vi "Check Posttrigger Countdown.vi"(8 "error in (no error)":errorcluster, 11 "Triggered Log in":refnum<class "Triggered Log.lvclass">) -> (0 "error out":errorcluster, 3 "Triggered Log out":refnum<class "Triggered Log.lvclass">)   [LabVIEW 2012, in "Triggered Log.lvclass"]
doc: "If the log is currently in the Posttrigger state, this VI checks the posttrigger countdown to see if it has reached zero. If so, this VI sets the triggered state of the log to either Waiting on Trigger or Complete based on whether the start trigger is retriggerable. It also notifies any listeners of the changed trigger state. Finally, if the posttrigger countdown is complete, this VI flushes any remaining data in the log buffer and closes the current file instance if specified."
uses:
  Triggered Log.lvclass
  Triggered Log.lvclass/Triggered Log.ctl
  Triggered Log State.ctl
  Engine/Classes/Logs/Segmented Logs/Segmented Log/Segmented Log.lvclass/Segmented Log.ctl
  Shared/Classes/Log File Specifications/Log File Specification/Log File Specification.lvclass/Log File Specification.ctl
  Flush Buffer Data to File.vi
  On Triggered Log State Change.vi
  Flush Buffer Data.vi
  Engine/Classes/Logs/Segmented Logs/Segmented Log/Write Data to Log File Instance (Waveform).vi
  Engine/Classes/Logs/Segmented Logs/Segmented Log/Write Data to Log File Instance.vi
  Engine/Classes/Logs/Segmented Logs/Segmented Log/Check Close File.vi
  Engine/Classes/Logs/Segmented Logs/Segmented Log/Check Open File.vi
  Engine/Classes/Logs/Segmented Logs/Segmented Log/Close Log File Instance.vi
  Engine/Classes/Logs/Segmented Logs/Segmented Log/Open Log File Instance.vi
  Engine/Classes/Logs/Segmented Logs/Segmented Log/On Segmented Log Complete.vi
  Engine/Classes/Logs/Segmented Logs/Segmented Log/On File Close.vi
  Shared/Classes/Log File Specifications/Log File Specification/Open Log File.vi
  Shared/Classes/Log File Specifications/Log File Specification/Set Path Tag.vi
  Engine/Classes/Logs/Segmented Logs/Segmented Log/On File Open.vi
  Shared/Classes/Log File Specifications/Log File Specification/Set Filename Offset.vi
  Shared/Classes/Log File Specifications/Log File Specification/Build File Path.vi
  Shared/Classes/Log File Specifications/Log File Specification/Resolve File Conflicts.vi
  Engine/Classes/Triggers/Trigger/Initialize.vi
  Engine/Classes/Triggers/Trigger/Finalize.vi
  Shared/Classes/Log File Specifications/Log File Specification/Initialize Log File.vi
  <vilib>/Utility/libraryn.llb/Check if File or Folder Exists.vi
  <vilib>/Utility/error.llb/Error Cluster From Error Code.vi
  <vilib>/Utility/libraryn.llb/Get File Extension.vi
  <vilib>/Utility/libraryn.llb/Create Directory Recursive.vi
  Engine/Classes/Logs/Log Files/Log File/Write to Log File (Waveform).vi
  Engine/Classes/Logs/Segmented Logs/Segmented Log/Segment Log File.vi
  Engine/Classes/Logs/Log Files/Log File/Close Log File.vi
  Engine/Classes/Logs/Segmented Logs/Segmented Log/Make File Read-Only.vi
  Engine/Classes/Logs/Log Files/Log File/Write to Log File.vi
  Engine/Classes/Logs/Log Files/Log File/Log File.lvclass
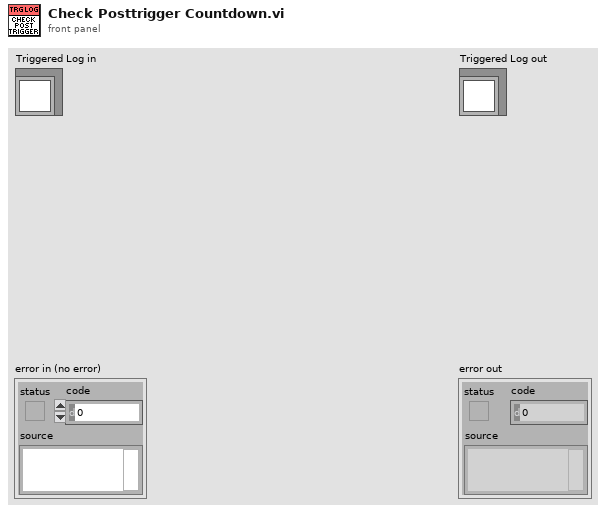
[diagram p1: front panel]
types:
  T1 = typedef "Triggered Log.lvclass/Triggered Log State.ctl" = enum16{"Waiting on Trigger", "Triggered", "Posttrigger", "Complete", "Idle", "Error"}
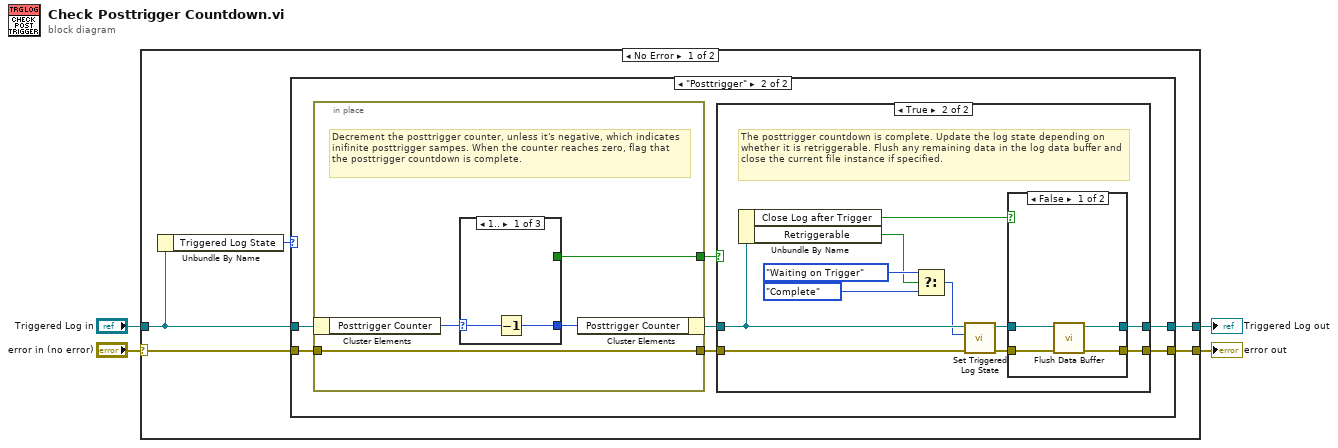
[diagram p0: block diagram]
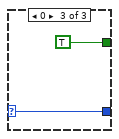
[diagram p4: hidden frame]
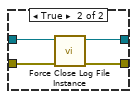
[diagram p6: hidden frame]
diagram:
  n1 = case shown="No Error" "error in (no error)" {
    selector: "error in (no error)" -> [w7 w50]
    tunnel: [w9 w50] -> w3
    tunnel: [w8 w49] -> w1
    tunnel: "Triggered Log in" -> [w6 w49]
    frame No Error {
      n2 = Unbundle By Name(w6) -> ("Triggered Log State"=w5:T1)
      n3 = case shown="\"Posttrigger\"" w5 {
        tunnel: [w10 w18] -> w9
        tunnel: [w11 w17] -> w8
        tunnel: w7 -> [w10 w12]
        tunnel: w6 -> [w11 w15]
        frame Default {
        }
        frame "Posttrigger" {
          n4 = in-place {
            in-place-border: [w22] -> w16
            in-place-border: [w19] -> w13
            in-place-border: w12 -> [w19]
            # "Decrement the posttrigger counter, unless it's negative, which indicates inifinite posttrigger sampes. When the counter reaches zero, flag that the posttrigger countdown is complete."
            n5 = in-place-cluster #1(w15) -> ("Posttrigger Counter"=w21:i64)
            n6 = case shown="1.." w21 {
              selector: w21 -> [w24 w25 w26]
              tunnel: [w23 w25 w26] -> w20
              tunnel: [_ _ TRUE] -> w22
              frame 1.. {
                n7 = Decrement(x=w24) -> (x-1=w23:i64)
              }
              frame ..-1 {
              }
              frame 0 {
              }
            }
            n8 = in-place-cluster #1("Posttrigger Counter"=w20) -> (w14:refnum<class "Triggered Log.lvclass">)
          }
          n9 = case shown="True" w16 {
            tunnel: w13 -> [w28 w34]
            tunnel: [w28 w40] -> w18
            tunnel: w14 -> [w29 w32]
            tunnel: [w29 w39] -> w17
            frame False {
            }
            frame True {
              # "The posttrigger countdown is complete. Update the log state depending on whether it is retriggerable. Flush any remaining data in the log data buffer and close the current file instance if specified."
              n10 = Unbundle By Name(w32) -> ("Close Log after Trigger"=w38:bool, "Retriggerable"=w35:bool)
              n11 = Select(t=Triggered_Log_State."Waiting on Trigger" ("Triggered Log State"), s=w35, f=Triggered_Log_State."Complete" ("Triggered Log State")) -> (s? t:f=w30:T1)
              n12 = call "Set Triggered Log State.vi"("error in (no error)"=w34, "Triggered Log State"=w30, "Triggered Log in"=w32) -> ("error out"=w33:errorcluster, "Triggered Log out"=w31:refnum<class "Triggered Log.lvclass">)  [unwired: 7 in]
              n13 = case shown="False" w38 {
                tunnel: w33 -> [w44 w48]
                tunnel: [w43 w47] -> w40
                tunnel: [w41 w46] -> w39
                tunnel: w31 -> [w42 w45]
                frame False {
                  n14 = call "Flush Data Buffer.vi"("error in (no error)"=w44, "Triggered Log in"=w42) -> ("error out"=w43:errorcluster, "Triggered Log out"=w41:refnum<class "Triggered Log.lvclass">)  [unwired: 8 in]
                }
                frame True {
                  n15 = call "Force Close Log File Instance.vi"("error in (no error)"=w48, "Triggered Log in"=w45) -> ("error out"=w47:errorcluster, "Triggered Log out"=w46:refnum<class "Triggered Log.lvclass">)  [unwired: 8 in]
                }
              }
            }
          }
        }
      }
    }
    frame Error {
    }
  }
  "error out" <- w3
  "Triggered Log out" <- w1
